vi "Target4.vi"() -> ()   [LabVIEW 2025]
uses:
  <vilib>/Platform/TimedLoop/XDataNode/timing_clust.ctl
  <vilib>/Platform/TimedLoop/XDataNode/nitl_modes.ctl
  <vilib>/Platform/TimedLoop/XDataNode/wakeup.ctl
  <vilib>/eio/utilities/niEioResolveVilibRelativePath.vi
  <vilib>/rvi/interface/RandomDataEmulation/niFpgaRandomDataHandleErrors.vi
  <vilib>/rvi/Emulation/niFpgaSctlEmulationGetInTimedLoop.vi
  <vilib>/rvi/Emulation/niFpgaEmulationReportErrorSimple.vi
  <vilib>/rvi/Emulation/niFpgaGetClockAttributes.vi
  <vilib>/rvi/Emulation/niFpgaCriticalErrorInLSC.vi
  <vilib>/rvi/linearAlgebra/MatrixMultiply/simVIs/SubVI/nifxpla_MatrixMultiply_SimMatrixSizes.vi
  <vilib>/rvi/linearAlgebra/MatrixMultiply/simVIs/SubVI/nifxpla_MatrixMultiply_Sim4WireAdapterVector.vi
  <vilib>/rvi/linearAlgebra/MatrixMultiply/simVIs/SubVI/nifxpla_MatrixMultiply_SimFrameHandShake.vi
  <vilib>/rvi/linearAlgebra/MatrixMultiply/simVIs/SubVI/nifxpla_MatrixMultiply_SimEndlessCounter.vi
  <vilib>/rvi/linearAlgebra/MatrixMultiply/simVIs/SubVI/nifxpla_MatrixMultiply_SimVectorDataBuffer.vi
  <vilib>/rvi/ClientSDK/Core/DevComputerLib/Private/Multiply(dfxp64).vi
  <vilib>/rvi/ClientSDK/Core/DevComputerLib/Private/Dfxp128ToDfxp256.vi
  <vilib>/rvi/ClientSDK/Core/DevComputerLib/Private/Add(dfxp256).vi
  <vilib>/rvi/ClientSDK/Core/DevComputerLib/Private/Subtract(dfxp256).vi
  <vilib>/rvi/ClientSDK/Core/DevComputerLib/Private/ToDfxp64(dfxp256).vi
  <vilib>/rvi/interface/RandomDataEmulation/nirviRandomDataMultiElementFPGAFIFO.vi
  <instcachedir>/0/nirviRandomDataMultiElementFPGAFIFO_BE2FF10D3D6E420AB0291A02835C249E.lvgen/nirviRandomDataMultiElementFPGAFIFO_BE2FF10D3D6E420AB0291A02835C249E_001.vi
  <vilib>/rvi/DataTransferAndStorage/Container/XNode/niFpgaContainer.xnode
  <vilib>/rvi/interface/RandomDataEmulation/nirviRandomDataFpgaReadWriteTemplate.vi
  <vilib>/platform/TimedLoop/XDataNode/XDataNode.xnode
  <vilib>/rvi/linearAlgebra/MatrixMultiply/XNode/nifxpla_MatrixMultiply.xnode
  <vilib>/rvi/linearAlgebra/MatrixMultiply/simVIs/nifxpla_MatrixMultiply_SimTemplateEinEout.vi
  <vilib>/rvi/linearAlgebra/MatrixMultiply/simVIs/nifxpla_MatrixMultiply_SimTemplateEinVout.vi
  <vilib>/rvi/linearAlgebra/MatrixMultiply/simVIs/nifxpla_MatrixMultiply_SimTemplateVinEout.vi
  <vilib>/rvi/linearAlgebra/MatrixMultiply/simVIs/nifxpla_MatrixMultiply_SimTemplateVinVout.vi
  <vilib>/rvi/interface/RandomDataEmulation/nirviRandomDataFpgaMultiElementTemplate.vi
  <vilib>/Platform/TimedLoop/XDataNode/XDNodeRunTimeDep.lvlib
panel:
  out "cr":fxp<+/-,32,16>[](array[numeric])
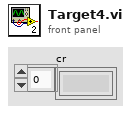
[diagram p1: front panel]
types:
  T1 = typedef "XDNodeRunTimeDep.lvlib/timing_clust.ctl" = cluster{"Expected End [f-1]":u64, "Actual End [f-1]":u64, "Finished Late? [f-1]":bool, "Expected End [i-1]":u64, "Actual End [i-1]":u64, "Finished Late? [i-1]":bool, "Expected Start [i]":u64, "Actual Start [i]":u64, "Expected Start [f]":u64, "Actual Start [f]":u64, "Source Name":string, "Structure Name":string, "Period":i64, "Deadline":i64, "Offset":i64, "Start":i64, "Priority":i32, "Timeout":i32, "Mode":T2, "Wakeup Reason":T3, "Error":errorcluster, "Source Type":string, "Secondary Source Type":string, "Global End Time":u64, "Global Start Time":u64, "Frame Duration":u64, "Iteration Duration":u64, "Assigned CPU":i32, "I/O Scan Engine Mode":u32}
  T2 = typedef "XDNodeRunTimeDep.lvlib/nitl_modes.ctl" = enum32{"No Change", "Process missed periods, maintain original phase", "Discard missed periods, maintain original phase", "Process missed periods, ignore original phase", "Discard missed periods, ignore original phase"}
  T3 = typedef "XDNodeRunTimeDep.lvlib/wakeup.ctl" = enum32{"Normal", "Aborted", "Asynchronous wakeup", "Timing source error", "Timed loop error", "Timeout"}
  T4 = cluster{"[0]":fxp<+/-,32,16>, "[1]":fxp<+/-,32,16>}
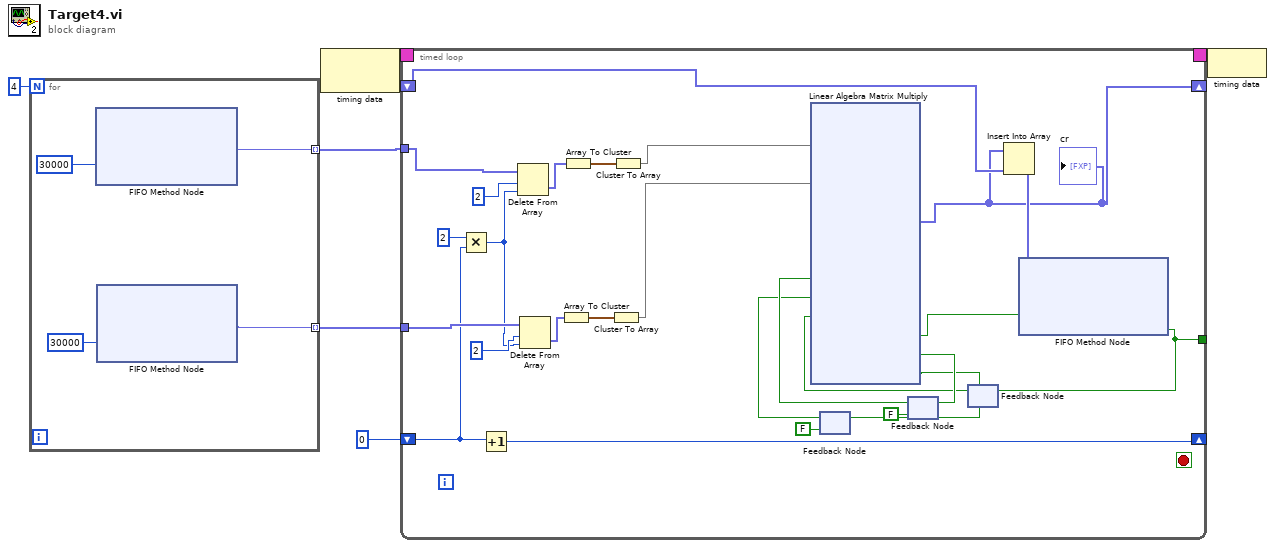
[diagram p0: block diagram]
diagram:
  n1 = for {
    N: 4 -> [_]
    tunnel: [w8] -> w2 mode=indexing
    tunnel: [w7] -> w3 mode=indexing
    n2 = xnode ("FIFO Method Node")("Timeout"=30000) -> ("Element"=w7:fxp<+/-,32,16>)  [unwired: 1 in, 2 out]
    n3 = xnode ("FIFO Method Node")("Timeout"=30000) -> ("Element"=w8:fxp<+/-,32,16>)  [unwired: 1 in, 2 out]
  }
  n4 = node-c288() -> (w6:T1)  [unwired: 1 in]
  n5 = timed-loop {
    timing: w6 -> [_]
    timing-out: [_] -> w5
    shift-right: [w26] -> _
    shift-left: _ -> [w27]
    tunnel: [w25] -> _
    tunnel: w3 -> [w24]
    tunnel: w2 -> [w22]
    shift-right: [w12] -> _
    shift-left: i16 0 -> [w11]
    stop <- _ stop-if-true
    n6 = Multiply(x=2, y=w11) -> (x*y=w13:i32)
    n7 = Increment(x=w11) -> (x+1=w12:i16)
    n8 = Delete From Array(array=w24, length=2, index=w13) -> (deleted portion=w20:fxp<+/-,32,16>[])  [unwired: 1 out]
    n9 = Delete From Array(array=w22, length=2, index=w13) -> (deleted portion=w18:fxp<+/-,32,16>[])  [unwired: 1 out]
    n10 = Array To Cluster(array=w18) -> (cluster=w17:T4)
    n11 = Array To Cluster(array=w20) -> (cluster=w19:T4)
    n12 = Cluster To Array(cluster=w17) -> (array=w21:fxp<+/-,32,16>[])
    n13 = Cluster To Array(cluster=w19) -> (array=w23:fxp<+/-,32,16>[])
    n14 = feedback #1(FALSE ("ready for b")) -> (w33:bool)
    n15 = feedback #2(FALSE ("ready for a")) -> (w35:bool)
    n16 = feedback #3() -> (w30:bool)  [unwired: 1 in]
    n17 = xnode ("Linear Algebra Matrix Multiply")("ar"=w23, "br"=w21, "a valid"=w35, "b valid"=w33, "ready for output (T)"=w30) -> ("cr"=w26:fxp<+/-,32,16>[], "output valid"=w29:bool, "ready for a"=w36:bool, "ready for b"=w34:bool)  [unwired: 2 in, 2 out]
    "cr" <- w26
    n18 = feedback-in #1(w34) -> ()
    n19 = feedback-in #2(w36) -> ()
    n20 = Insert Into Array(array=w26, new element=w27) -> (w28:fxp<+/-,32,16>[])  [unwired: 1 in]
    n21 = xnode ("FIFO Method Node")("Element"=w28, "Input Valid"=w29) -> ("Ready for Input"=w25:bool)  [unwired: 1 in, 1 out]
    n22 = feedback-in #3(w25) -> ()
  }
  n23 = node-c288(w5) -> ()
